vi "save_infos_v3_svi.vi"(0 "Refnum VISA en entrée":refnum<visa-resource-name>, 1 "Non 2":u32, 2 "ROMODE":u32, 3 "Nstart 2":u32, 4 "SOFT_VERSION":string, 5 "Noff":u32, 6 "Camera Model":string, 8 "BIN":u16, 9 "Non":u32, 10 "Noff 2":u32, 11 "Camera Serial":string, 12 "EXPT":dbl, 13 "Version":string, 14 "USED_FILTERS":u8[](array[numeric]), 15 "STAGE_SPEED":dbl, 16 "info Directory":path, 17 "NSCAN":u32, 18 "USED_LEDS":bool[][](array[boolean]), 19 "BETWEEN_SCAN":u32, 25 "Nstart":u32, 26 "BETWEEN_PAT":u32, 27 "NPAT":u32) -> ()   [LabVIEW 2013]
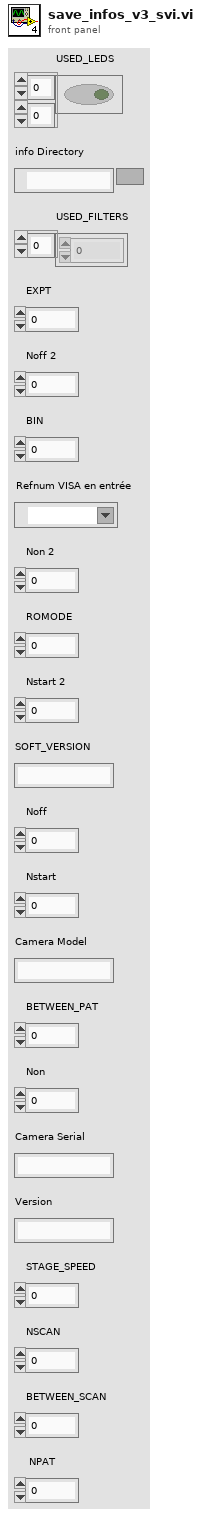
[diagram p1: front panel]
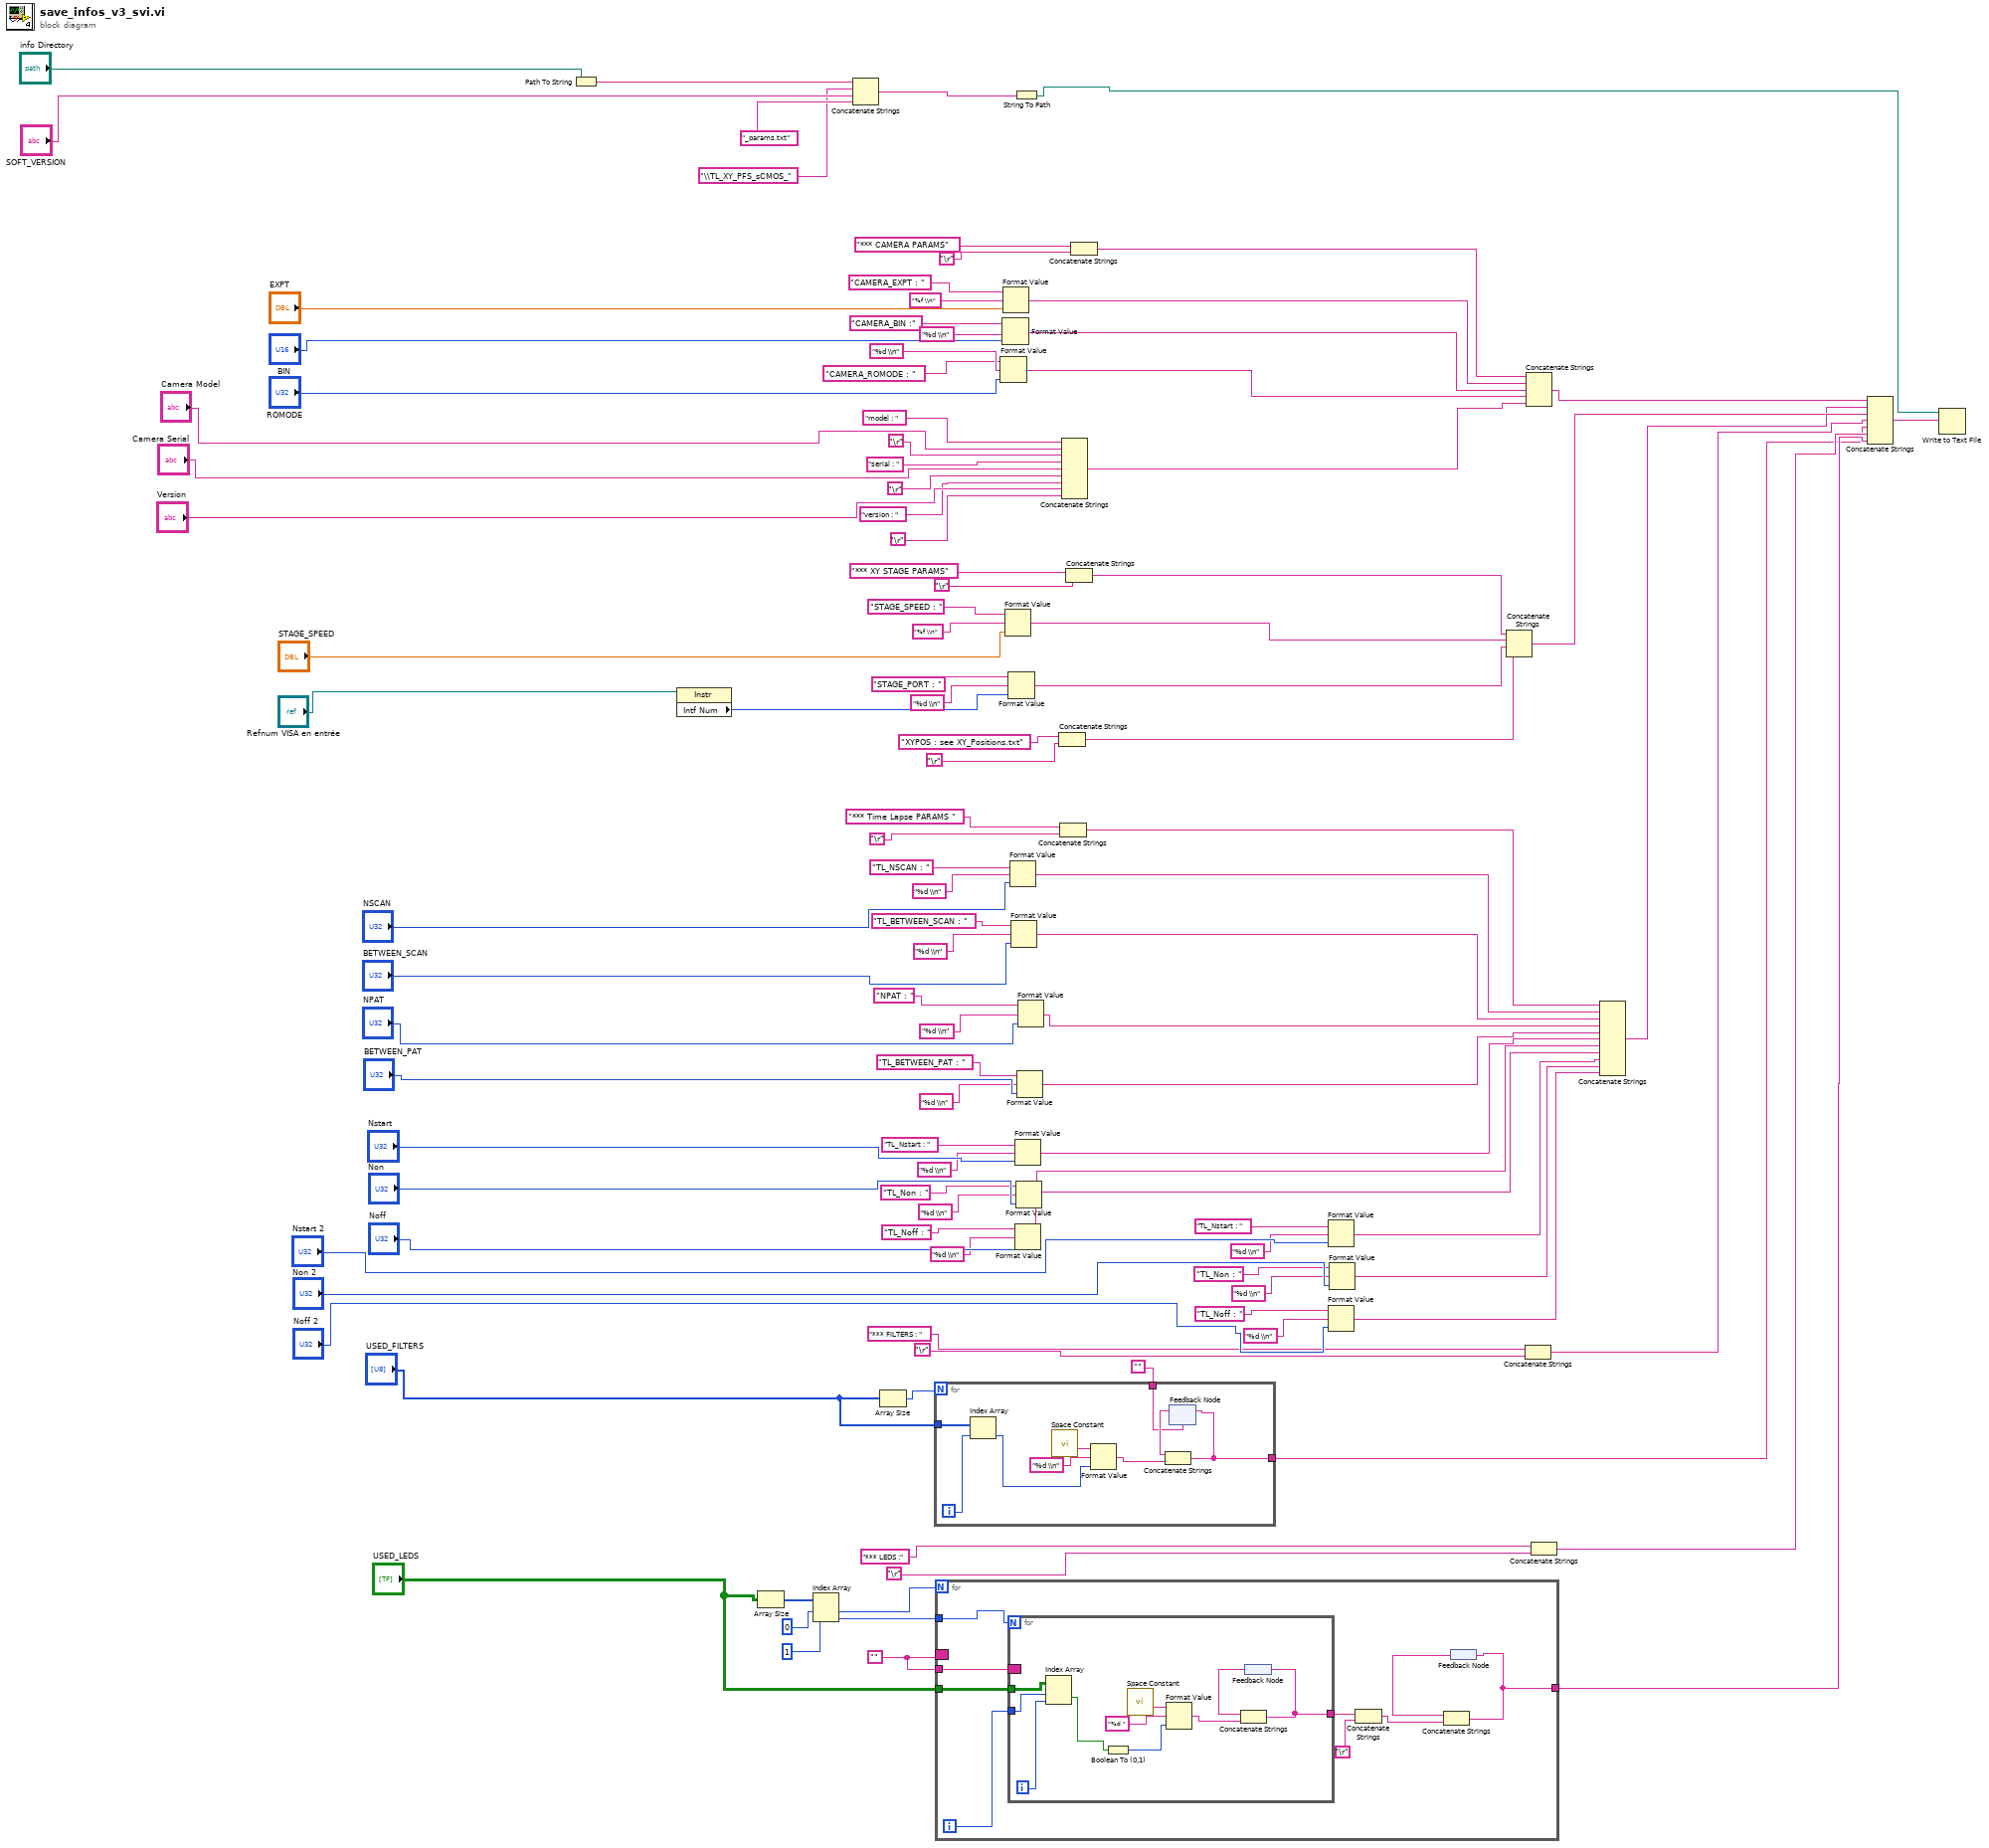
[diagram p0: block diagram]
diagram:
  w100 = ""
  n1 = Path To String(path="info Directory") -> (string=w2:string)
  n2 = property class="Instr"(reference="Refnum VISA en entrée") -> ("Intf Num"=w27:u16)  [unwired: 1 in, 2 out]
  n3 = Array Size(array="USED_LEDS") -> (size(s)=w66:i32[])
  n4 = Index Array(array=w66, index #1=0, index #2=1) -> (element #1=w67:i32, element #2=w99:i32)
  n5 = Concatenate Strings(w2, "\\TL_XY_PFS_sCMOS_", "SOFT_VERSION", "_params.txt") -> (w6:string)
  n6 = Array Size(array="USED_FILTERS") -> (size(s)=w61:i32)
  n7 = for {
    N: w61 -> [_]
    tunnel: "USED_FILTERS" -> [w118]
    tunnel: "" -> [w114]
    tunnel: [w113] -> w90
    i -> [w119]
    n8 = Index Array(array=w118, index=w119) -> (element=w117:u8)
    n9 = call <vilib>:"Space Constant.vi"() -> ("String"=w120:string)
    n10 = Format Value(string ("")=w120, format string="%d \\n", value (0)=w117) -> (output string=w116:string)
    n11 = feedback #1(w114) -> (w115:string)
    n12 = Concatenate Strings(w115, w116) -> (w113:string)
    n13 = feedback-in #1(w113) -> ()
  }
  n14 = for {
    N: w67 -> [_]
    tunnel: "USED_LEDS" -> [w130]
    tunnel: [w124] -> w92
    tunnel: w99 -> [w123]
    border: w100 -> [_]
    tunnel: w100 -> [w122]
    i -> [w129]
    n15 = for {
      N: w123 -> [_]
      tunnel: w130 -> [w139]
      tunnel: w129 -> [w131]
      tunnel: [w133] -> w127
      border: w122 -> [_]
      i -> [w132]
      n16 = Index Array(array=w139, index (row)=w131, index (col)=w132) -> (element=w137:bool)
      n17 = Boolean To (0,1)(Boolean=w137) -> (0, 1=w136:i16)
      n18 = call <vilib>:"Space Constant.vi"() -> ("String"=w138:string)
      n19 = Format Value(string ("")=w138, format string="%d ", value (0)=w136) -> (output string=w135:string)
      n20 = feedback #2() -> (w134:string)
      n21 = Concatenate Strings(w134, w135) -> (w133:string)
      n22 = feedback-in #2(w133) -> ()
    }
    n23 = Concatenate Strings(w127, "\r") -> (w126:string)
    n24 = feedback #3() -> (w125:string)
    n25 = Concatenate Strings(w125, w126) -> (w124:string)
    n26 = feedback-in #3(w124) -> ()
  }
  n27 = Format Value(string ("")="CAMERA_ROMODE : ", format string="%d \\n", value (0)="ROMODE") -> (output string=w84:string)
  n28 = Format Value(string ("")="CAMERA_BIN :", format string="%d \\n", value (0)="BIN") -> (output string=w83:string)
  n29 = Format Value(string ("")="CAMERA_EXPT : ", format string="%f \\n", value (0)="EXPT") -> (output string=w82:string)
  n30 = Format Value(string ("")="STAGE_SPEED : ", format string="%f \\n", value (0)="STAGE_SPEED") -> (output string=w79:string)
  n31 = Format Value(string ("")="STAGE_PORT : ", format string="%d \\n", value (0)=w27) -> (output string=w80:string)
  n32 = Format Value(string ("")="TL_NSCAN : ", format string="%d \\n", value (0)="NSCAN") -> (output string=w71:string)
  n33 = Format Value(string ("")="TL_BETWEEN_SCAN : ", format string="%d \\n", value (0)="BETWEEN_SCAN") -> (output string=w72:string)
  n34 = String To Path(string=w6) -> (path=w94:path)
  n35 = Format Value(string ("")="TL_Nstart : ", format string="%d \\n", value (0)="Nstart") -> (output string=w75:string)
  n36 = Format Value(string ("")="TL_Noff : ", format string="%d \\n", value (0)="Noff") -> (output string=w77:string)
  n37 = Format Value(string ("")="TL_Non : ", format string="%d \\n", value (0)="Non") -> (output string=w76:string)
  n38 = Format Value(string ("")="TL_BETWEEN_PAT : ", format string="%d \\n", value (0)="BETWEEN_PAT") -> (output string=w74:string)
  n39 = Format Value(string ("")="NPAT : ", format string="%d \\n", value (0)="NPAT") -> (output string=w73:string)
  n40 = Concatenate Strings("XYPOS : see XY_Positions.txt", "\r") -> (w97:string)
  n41 = Concatenate Strings("*** Time Lapse PARAMS ", "\r") -> (w70:string)
  n42 = Concatenate Strings("model : ", "Camera Model", "\r", "serial : ", "Camera Serial", "\r", "version : ", "Version", "\r") -> (w85:string)
  n43 = Concatenate Strings("*** XY STAGE PARAMS", "\r") -> (w78:string)
  n44 = Concatenate Strings("*** CAMERA PARAMS", "\r") -> (w81:string)
  n45 = Format Value(string ("")="TL_Nstart : ", format string="%d \\n", value (0)="Nstart 2") -> (output string=w110:string)
  n46 = Format Value(string ("")="TL_Noff : ", format string="%d \\n", value (0)="Noff 2") -> (output string=w112:string)
  n47 = Format Value(string ("")="TL_Non : ", format string="%d \\n", value (0)="Non 2") -> (output string=w111:string)
  n48 = Concatenate Strings(w78, w79, w80, w97) -> (w87:string)
  n49 = Concatenate Strings("*** FILTERS : ", "\r") -> (w89:string)
  n50 = Concatenate Strings(w81, w82, w83, w84, w85) -> (w86:string)
  n51 = Concatenate Strings("*** LEDS :", "\r") -> (w91:string)
  n52 = Concatenate Strings(w70, w71, w72, w73, w74, w75, w76, w77, w110, w111, w112) -> (w88:string)
  n53 = Concatenate Strings(w86, w87, w88, w89, w90, w91, w92) -> (w93:string)
  n54 = Write to Text File(file (use dialog)=w94, text=w93) -> ()  [unwired: 2 in, 3 out]
